vi "LakeShore 336 Read.vi"(4 "error in (no error)":errorcluster, 5 "Point #":i32, 6 "Parameters":dbl[](array[numeric]) format="%.3e", 7 "Instrument Address":refnum<visa-resource-name>) -> (0 "Error Out":errorcluster, 1 "Stop":bool, 2 "Measurement":dbl[](array[numeric]) format="%.6e", 3 "dup VISA session":refnum<visa-resource-name>)   [LabVIEW 2025]
doc: "This VI reads a single reading from a LakeShore 340 Temperature Controller. The stop boolean is always false. If no reading is obtained a single zero is returned.\nParameter 0 - 0=Resistance, 1=Temperature, 2=Heater Power\nParameter 1 - Channel to read, channel 0 is channel A, etc.\nScott Hannahs, <sth@magnet.fsu.edu> NHMFL-FSU, May 2003\nAuthor: Scott Hannahs <sth@magnet.fsu.edu>\n\nThis software is licensed for use under the “MIT License\"\nCopyright (c) 2025 Scott Hannahs, sth@sth@magnet.sthnet.net\n\nPermission is hereby granted, free of charge, to any person obtaining a copy of this software and associated documentation files (the \"Software\"), to deal in the Software without restriction, including without limitation the rights to use, copy, modify, merge, publish, distribute, sublicense, and/or sell copies of the Software, and to permit persons to whom the Software is furnished to do so, subject to the following conditions: The above copyright notice and this permission notice shall be included in all copies or substantial portions of the Software.\n\nTHE SOFTWARE IS PROVIDED \"AS IS\", WITHOUT WARRANTY OF ANY KIND, EXPRESS OR IMPLIED, INCLUDING BUT NOT LIMITED TO THE WARRANTIES OF MERCHANTABILITY, FITNESS FOR A PARTICULAR PURPOSE AND NONINFRINGEMENT. IN NO EVENT SHALL THE AUTHORS OR COPYRIGHT HOLDERS BE LIABLE FOR ANY CLAIM, DAMAGES OR OTHER LIABILITY, WHETHER IN AN ACTION OF CONTRACT, TORT OR OTHERWISE, ARISING FROM, OUT OF OR IN CONNECTION WITH THE SOFTWARE OR THE USE OR OTHER DEALINGS IN THE SOFTWARE."
panel:
  # "The first parameter tells it\nHeater power if =2\nto read temperature if =1\nResistance if =0\nThe second is channel #"
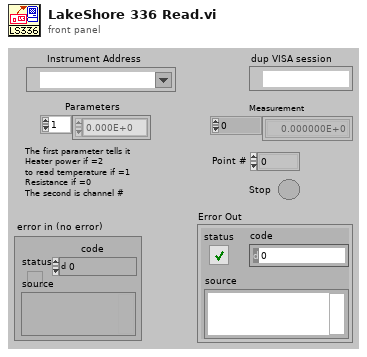
[diagram p1: front panel]
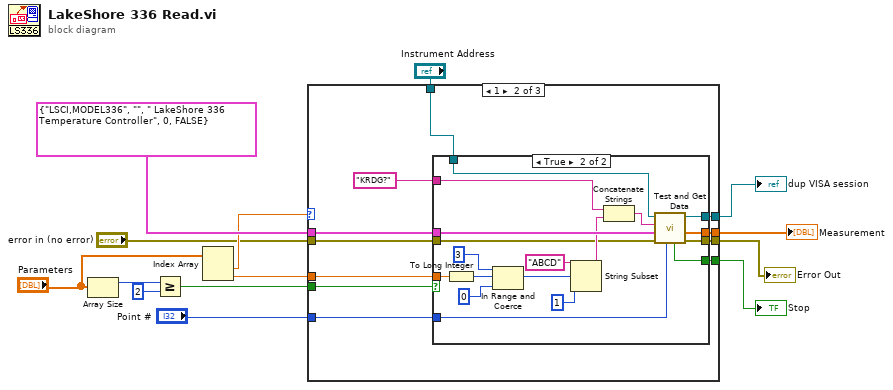
[diagram p0: block diagram]
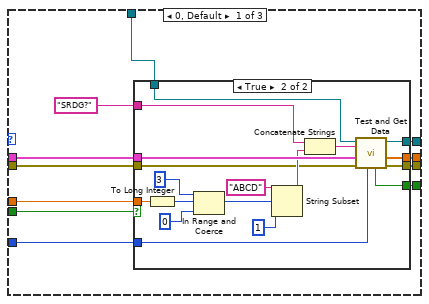
[diagram p2: hidden frame]
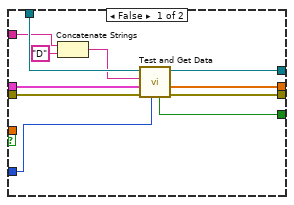
[diagram p3: hidden frame]
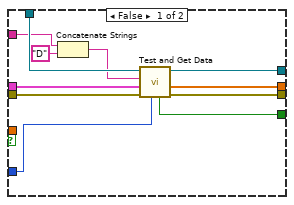
[diagram p4: hidden frame]
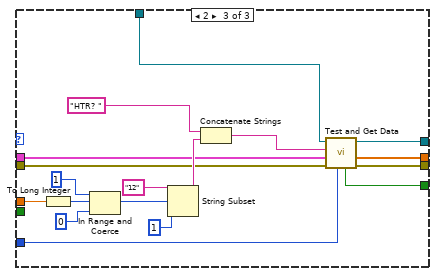
[diagram p5: hidden frame]
diagram:
  n1 = Array Size(array="Parameters") -> (size(s)=w8:i32)
  n2 = Greater Or Equal?(x=w8, y=2) -> (x >= y?=w11:bool)
  n3 = Index Array(array="Parameters") -> (element #1=w4:dbl, element #2=w6:dbl)  [unwired: 2 in]
  n4 = case shown="1" w4 {
    tunnel: cluster{string, string, string, u32, bool} {"LSCI,MODEL336", "", " LakeShore 336 Temperature Controller", 0, FALSE} -> [w25 w65 w97]
    tunnel: [w24 w64 w101] -> w13
    tunnel: [w23 w63 w95] -> w12
    tunnel: w11 -> [w22 w62 _]
    tunnel: "Point #" -> [w21 w61 w96]
    tunnel: w6 -> [w20 w60 w112]
    tunnel: "Instrument Address" -> [w19 w59 w102]
    tunnel: [w15 w55 w99] -> w1
    tunnel: "error in (no error)" -> [w17 w57 w98]
    tunnel: [w16 w56 w100] -> w2
    frame 0, Default {
      n5 = case shown="True" w22 {
        tunnel: w25 -> [w36 w51]
        tunnel: w19 -> [w35 w54]
        tunnel: [w31 w50] -> w24
        tunnel: [w27 w39] -> w23
        tunnel: w21 -> [w34 w53]
        tunnel: w20 -> [_ w46]
        tunnel: "SRDG?" ("Format String") -> [w29 w45]
        tunnel: w17 -> [w33 w38]
        tunnel: [w32 w40] -> w16
        tunnel: [w26 w37] -> w15
        frame False {
          n6 = Concatenate Strings(w29, "D" ("string")) -> (w28:string)
          n7 = call "Test and Get Data.vi"("Point #"=w34, "error in (no error)"=w33, "Instrument Info"=w36, "Command String"=w28, "VISA Sesson"=w35) -> ("Error Out"=w26:errorcluster, "Measurement"=w31:dbl[], "dup VISA session"=w32:refnum<visa-resource-name>, "Stop"=w27:bool)  [unwired: 1 in, 1 out]
        }
        frame True {
          n8 = To Long Integer(number=w46) -> (32bit integer=w47:i32)
          n9 = In Range and Coerce(upper limit=3, x=w47, lower limit=0) -> (coerced(x)=w42:i32)  [unwired: 1 out]
          n10 = String Subset(string="ABCD", offset (0)=w42, length (rest)=1 ("length (rest)")) -> (substring=w41:string)
          n11 = Concatenate Strings(w45, w41) -> (w52:string)
          n12 = call "Test and Get Data.vi"("Point #"=w53, "error in (no error)"=w38, "Instrument Info"=w51, "Command String"=w52, "VISA Sesson"=w54) -> ("Error Out"=w37:errorcluster, "Measurement"=w50:dbl[], "dup VISA session"=w40:refnum<visa-resource-name>, "Stop"=w39:bool)  [unwired: 1 in, 1 out]
        }
      }
    }
    frame 1 {
      n13 = case shown="True" w62 {
        tunnel: w65 -> [w76 w91]
        tunnel: w59 -> [w75 w94]
        tunnel: [w71 w90] -> w64
        tunnel: [w67 w77] -> w63
        tunnel: w61 -> [w74 w93]
        tunnel: w60 -> [_ w86]
        tunnel: "KRDG?" ("Format String") -> [w69 w85]
        tunnel: w57 -> [w73 w79]
        tunnel: [w72 w80] -> w56
        tunnel: [w66 w78] -> w55
        frame False {
          n14 = Concatenate Strings(w69, "D" ("string")) -> (w68:string)
          n15 = call "Test and Get Data.vi"("Point #"=w74, "error in (no error)"=w73, "Instrument Info"=w76, "Command String"=w68, "VISA Sesson"=w75) -> ("Error Out"=w66:errorcluster, "Measurement"=w71:dbl[], "dup VISA session"=w72:refnum<visa-resource-name>, "Stop"=w67:bool)  [unwired: 1 in, 1 out]
        }
        frame True {
          n16 = To Long Integer(number=w86) -> (32bit integer=w87:i32)
          n17 = In Range and Coerce(upper limit=3, x=w87, lower limit=0) -> (coerced(x)=w82:i32)  [unwired: 1 out]
          n18 = String Subset(string="ABCD", offset (0)=w82, length (rest)=1 ("length (rest)")) -> (substring=w81:string)
          n19 = Concatenate Strings(w85, w81) -> (w92:string)
          n20 = call "Test and Get Data.vi"("Point #"=w93, "error in (no error)"=w79, "Instrument Info"=w91, "Command String"=w92, "VISA Sesson"=w94) -> ("Error Out"=w78:errorcluster, "Measurement"=w90:dbl[], "dup VISA session"=w80:refnum<visa-resource-name>, "Stop"=w77:bool)  [unwired: 1 in, 1 out]
        }
      }
    }
    frame 2 {
      n21 = To Long Integer(number=w112) -> (32bit integer=w108:i32)
      n22 = In Range and Coerce(upper limit=1, x=w108, lower limit=0) -> (coerced(x)=w105:i32)  [unwired: 1 out]
      n23 = String Subset(string="12", offset (0)=w105, length (rest)=1 ("length (rest)")) -> (substring=w104:string)
      n24 = Concatenate Strings("HTR? " ("Format String"), w104) -> (w103:string)
      n25 = call "Test and Get Data.vi"("Point #"=w96, "error in (no error)"=w98, "Instrument Info"=w97, "Command String"=w103, "VISA Sesson"=w102) -> ("Error Out"=w99:errorcluster, "Measurement"=w101:dbl[], "dup VISA session"=w100:refnum<visa-resource-name>, "Stop"=w95:bool)  [unwired: 1 in, 1 out]
    }
  }
  "Stop" <- w12
  "Measurement" <- w13
  "dup VISA session" <- w2
  "Error Out" <- w1
